vi "TestHemisphere.vi"() -> ()   [LabVIEW 2013]
uses:
  Data/TypeDefs/UTM Location.ctl
  <vilib>/myRIO/Common/Instrument Driver Framework/myRIO v1.0/UART/vis/myRIO v1.0 Close UART.vi
  <vilib>/myRIO/Common/Instrument Driver Framework/Utilities/vis/FPGA Ref Manager.vi
  <vilib>/myRIO/Common/Instrument Driver Framework/myRIO v1.0/myRIO v1.0 Reset FPGA.vi
  <vilib>/myRIO/Instrument Drivers/Utilities/Utilities.lvlib
panel:
  out "Bytes at Port":u32
  out "Flow":u16(ring) items=["None", "XON/XOFF", "RTS/CTS", "XON/XOFF & RTS/CTS", "DTR/DSR", "XON/XOFF & DTR/DSR"]
  out "Parity":u16(ring) items=["None", "Odd", "Even", "Mark", "Space"]
  out "Baud Rate":u32
  out "Raw string":string
  out "VISA read buffer":string
  out "Stop  Button\nHeartbeat":bool
  out "Stop Button\nLoop modulo":i32
  out "Read loop counter":i32
  out "Heartbeat":bool
  out "Roll":dbl
  out "Pitch":dbl
  out "Boat Speed":dbl
  out "Boat Direction":dbl
  out "Boat Location":T1 {"North" format="%#_10f"; "East" format="%#_8f"}
  in  "stop":bool
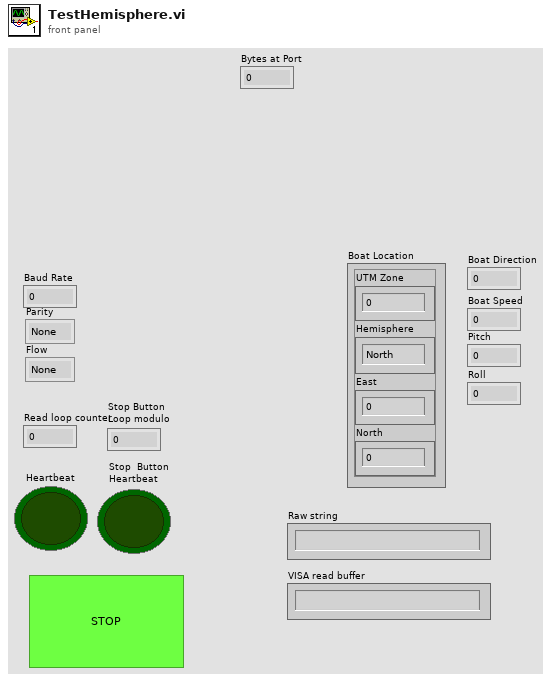
[diagram p1: front panel]
types:
  T1 = typedef "UTM Location.ctl" = cluster{"UTM Zone":dbl, "Hemisphere":enum16{"North", "South"}, "East":dbl, "North":dbl}
  T2 = typedef "Notifiers.ctl" = cluster{"BoatSpeed":refnum<notifier>, "WindSpeed":refnum<notifier>, "MissionCheckOff":refnum<notifier>, "EStop":refnum<notifier>, "SpeedOverWater":refnum<notifier>, "BoatDirection":refnum<notifier>, "Luffing":refnum<notifier>, "RudderForce":refnum<notifier>, "BatteryVoltage":refnum<notifier>, "StayForces":refnum<notifier>, "BoatLocation":refnum<notifier>, "Pitch":refnum<notifier>, "Roll":refnum<notifier>, "RateOfTurn":refnum<notifier>, "RelWindDirection":refnum<notifier>, "SailPositions":refnum<notifier>, "RudderPosition":refnum<notifier>, "IronsRange":refnum<notifier>, "AbsWindDirection":refnum<notifier>, "OverrideInformation":refnum<notifier>, "DynamixelTorques":refnum<notifier>, "MotorSetup":refnum<notifier>, "Airmar Status":refnum<notifier>, "HardwareOnline?":refnum<notifier>, "Sim_ActualSailPositions [0,1]":refnum<notifier>, "DynamixelCycleTracker":refnum<notifier>, "BoatVelocityDirection":refnum<notifier>, "Sim_Wind_Heading (rad)":refnum<notifier>, "Sim_Wind_Speed (m/s)":refnum<notifier>}
  T3 = typedef "GPS-Compass Queue Cluster.ctl" = cluster{"BoatLocation Queue":refnum<queue>, "BoatDirection Queue":refnum<queue>, "BoatSpeed Queue":refnum<queue>, "RateOfTurn Queue":refnum<queue>, "Pitch Queue":refnum<queue>, "Roll Queue":refnum<queue>, "BoatVelocityDirection Queue ":refnum<queue>}
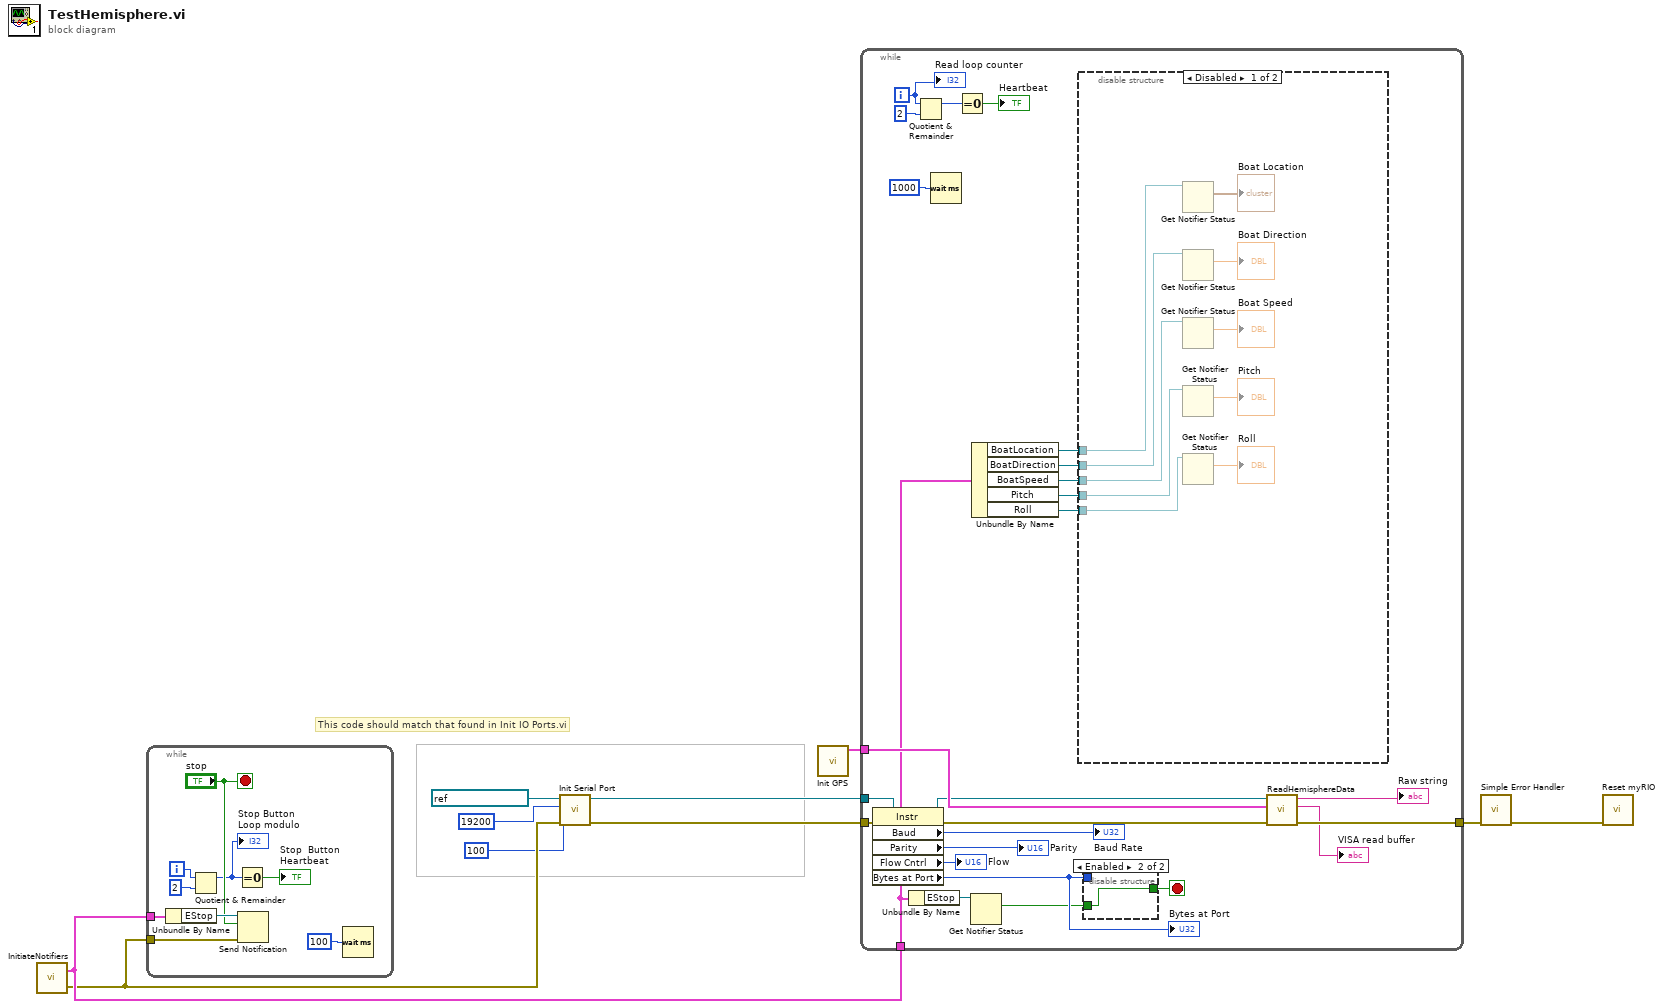
[diagram p0: block diagram]
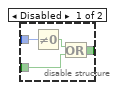
[diagram p2: hidden frame]
diagram:
  # "This code should match that found in Init IO Ports.vi"
  n1 = call "InitiateNotifiers.vi"() -> ("error out"=w2:errorcluster, "NotifierReferences"=w7:T2)  [unwired: 2 in]
  n2 = while {
    tunnel: w7 -> [w17]
    tunnel: w2 -> [w11]
    i -> [w13]
    stop <- "stop" stop-if-true
    n3 = Unbundle By Name(w17) -> ("EStop"=w18:refnum<notifier>)
    n4 = Quotient & Remainder(x=w13, y=2) -> (x-y*floor(x/y)=w12:i32)  [unwired: 1 out]
    "Stop Button\nLoop modulo" <- w12
    n5 = Equal To 0?(x=w12) -> (x = 0?=→"Stop  Button\nHeartbeat":bool)
    n6 = Send Notification(notification="stop", notifier=w18, error in (no error)=w11) -> ()  [unwired: 2 out]
    n7 = Wait (ms)(milliseconds to wait=u32 100) -> ()  [unwired: 1 out]
  }
  n8 = call "Init Serial Port.vi"("error in (no error)"=w2, "Input\nbuffer size"=u32 100 ("Input\nbuffer size"), "baud rate"=u32 19200, "VISA Refnum in"=refnum<visa-resource-name> "ASRL1::INSTR") -> ("error out"=w5:errorcluster, "VISA Refnum out"=w6:refnum<visa-resource-name>)  [unwired: 6 in]
  n9 = call "Init GPS.vi"() -> ("GPS-Compass Queue Cluster"=w10:T3)  [unwired: 11 in]
  n10 = while {
    tunnel: w10 -> [w43]
    tunnel: w7 -> [w32]
    tunnel: [w35] -> w9
    tunnel: w6 -> [w27]
    tunnel: w5 -> [w33]
    i -> [w29]
    stop <- w21 stop-if-true
    n11 = property class="Instr"(reference=w27) -> (reference out=w26:refnum<visa-resource-name>, "Baud"=→"Baud Rate":u32, "Parity"=→"Parity":u16, "Flow Cntrl"=→"Flow":u16, "Bytes at Port"=w22:u32)  [unwired: 1 in, 1 out]
    "Bytes at Port" <- w22
    n12 = Unbundle By Name(w32) -> ("EStop"=w31:refnum<notifier>)
    n13 = Quotient & Remainder(x=w29, y=2) -> (x-y*floor(x/y)=w34:i32)  [unwired: 1 out]
    n14 = Wait (ms)(milliseconds to wait=u32 1000) -> ()  [unwired: 1 out]
    n15 = Equal To 0?(x=w34) -> (x = 0?=→"Heartbeat":bool)
    n16 = Get Notifier Status(notifier=w31) -> (current notification=w20:bool)  [unwired: 1 in, 4 out]
    n17 = Unbundle By Name(w32) -> ("BoatLocation"=w42:refnum<notifier>, "BoatDirection"=w41:refnum<notifier>, "BoatSpeed"=w40:refnum<notifier>, "Pitch"=w39:refnum<notifier>, "Roll"=w38:refnum<notifier>)
    n18 = disable-structure shown="Disabled" {
      disable-tunnel: w42 -> [w59 _]
      disable-tunnel: w41 -> [w58 _]
      disable-tunnel: w40 -> [w57 _]
      disable-tunnel: w39 -> [w56 _]
      disable-tunnel: w38 -> [w55 _]
      frame Disabled {
        n19 = Get Notifier Status(notifier=w59) -> (current notification=→"Boat Location":T1)  [unwired: 1 in, 4 out]
        n20 = Get Notifier Status(notifier=w58) -> (current notification=→"Boat Direction":dbl)  [unwired: 1 in, 4 out]
        n21 = Get Notifier Status(notifier=w57) -> (current notification=→"Boat Speed":dbl)  [unwired: 1 in, 4 out]
        n22 = Get Notifier Status(notifier=w56) -> (current notification=→"Pitch":dbl)  [unwired: 1 in, 4 out]
        n23 = Get Notifier Status(notifier=w55) -> (current notification=→"Roll":dbl)  [unwired: 1 in, 4 out]
      }
      frame Enabled {
      }
    }
    n24 = disable-structure shown="Enabled" {
      disable-tunnel: w22 -> [w48 _]
      disable-tunnel: [w46 w49] -> w21
      disable-tunnel: w20 -> [w45 w49]
      frame Disabled {
        n25 = Not Equal To 0?(x=w48) -> (x != 0?=w47:bool)
        n26 = Or(x=w47, y=w45) -> (x .or. y?=w46:bool)
      }
      frame Enabled {
      }
    }
    n27 = call "ReadHemisphereData.vi"("Error in"=w33, "Hemisphere Queue Cluster"=w43, "VISA UART port"=w26) -> ("Error out"=w35:errorcluster, "Sentence"=→"VISA read buffer":string, "Raw string"=→"Raw string":string)  [unwired: 6 in]
    "Read loop counter" <- w29
  }
  n28 = call <vilib>:"Simple Error Handler.vi"("error in (no error)"=w9) -> ("error out"=w8:errorcluster)  [unwired: 4 in, 4 out]
  n29 = call <vilib>:"Reset myRIO.vi"("error in (no error)"=w8) -> ()  [unwired: 10 in, 1 out]
